vi "ClientFirstBare.vi"(8 "error in (no error)":errorcluster, 11 "WampScramAuthenticator in":refnum<class "WampScramAuthenticator.lvclass">) -> (0 "error out":errorcluster, 2 "ClientFirstBare":string, 3 "WampScramAuthenticator out":refnum<class "WampScramAuthenticator.lvclass">)   [LabVIEW 2020, in "wamplv.lvlib" / "WampScramAuthenticator.lvclass"]
uses:
  WampScramAuthenticator.lvclass
  WampScramAuthenticator.lvclass/WampScramAuthenticator.ctl
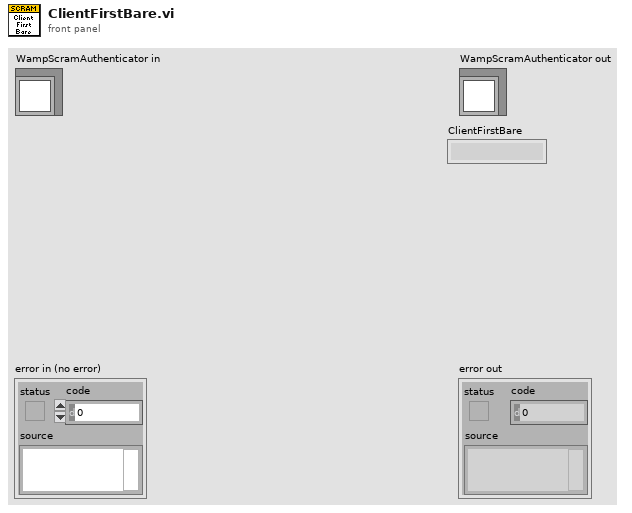
[diagram p1: front panel]
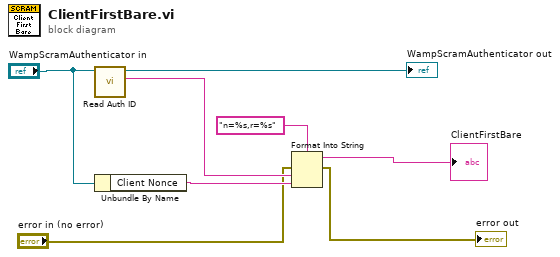
[diagram p0: block diagram]
diagram:
  n1 = call-dynamic "Read Auth ID.vi"("SecretBasedAuthenticatorBase in"="WampScramAuthenticator in") -> ("Auth ID"=w7:string, "SecretBasedAuthenticatorBase out"=→"WampScramAuthenticator out":refnum<class "WampScramAuthenticator.lvclass">)  [unwired: 8 in, 1 out]
  n2 = Unbundle By Name("WampScramAuthenticator in") -> ("Client Nonce"=w5:string)
  n3 = Format Into String(format string="n=%s,r=%s", error in="error in (no error)", w7, w5) -> (resulting string=→"ClientFirstBare":string, error out=→"error out":errorcluster)  [unwired: 1 in]
